vi "Init Root Actors.vi"(6 "Core Actors":refnum<class "Actor.lvclass">[](array[class]), 9 "Mid Actors":refnum<class "Actor.lvclass">[](array[class]), 10 "Edge Actors":refnum<class "Actor.lvclass">[](array[class])) -> (3 "Base Root Actors out":refnum<class "Base Root Actors.lvclass">)   [LabVIEW 2020, in "jettl.lvlib" / "Base Root Actors.lvlib" / "Base Root Actors.lvclass"]
uses:
  Base Root Actors.lvclass
  Actor/Actor.lvclass
  Base Root Actors.lvclass/Base Root Actors.ctl
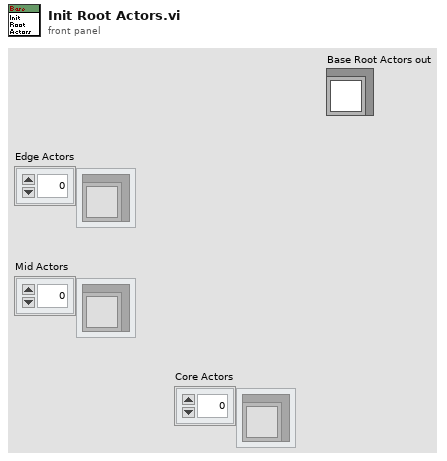
[diagram p1: front panel]
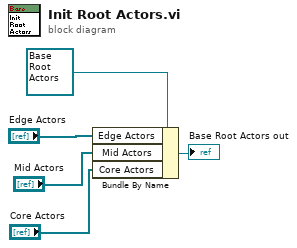
[diagram p0: block diagram]
diagram:
  n1 = Bundle By Name(cluster=refnum<class "Base Root Actors.lvclass"> refnum ("Base Root Actors out"), "Edge Actors"="Edge Actors", "Mid Actors"="Mid Actors", "Core Actors"="Core Actors") -> (→"Base Root Actors out":refnum<class "Base Root Actors.lvclass">)
